vi "UI.vi"() -> ()   [LabVIEW 2015]
panel:
  out "Input Registers 7":u16
  out "Input Registers 6":u16
  out "Input Registers 5":u16
  out "Input Registers 4":u16
  out "Input Registers 3":u16
  out "Input Registers 2":u16
  out "Input Registers 1":u16
  out "Input Registers 0":u16
  in  "Holding Registers 7":u16
  in  "Holding Registers 6":u16
  in  "Holding Registers 5":u16
  in  "Holding Registers 4":u16
  in  "Holding Registers 3":u16
  in  "Holding Registers 2":u16
  in  "Holding Registers 1":u16
  in  "Holding Registers 0":u16
  out "Discrete Inputs 7":bool
  out "Discrete Inputs 6":bool
  out "Discrete Inputs 5":bool
  out "Discrete Inputs 4":bool
  out "Discrete Inputs 3":bool
  out "Discrete Inputs 2":bool
  out "Discrete Inputs 1":bool
  in  "Coils 7":bool
  in  "Coils 6":bool
  in  "Coils 5":bool
  in  "Coils 4":bool
  in  "Coils 3":bool
  in  "Coils 2":bool
  in  "Coils 1":bool
  out "Discrete Inputs 0":bool
  in  "Coils 0":bool
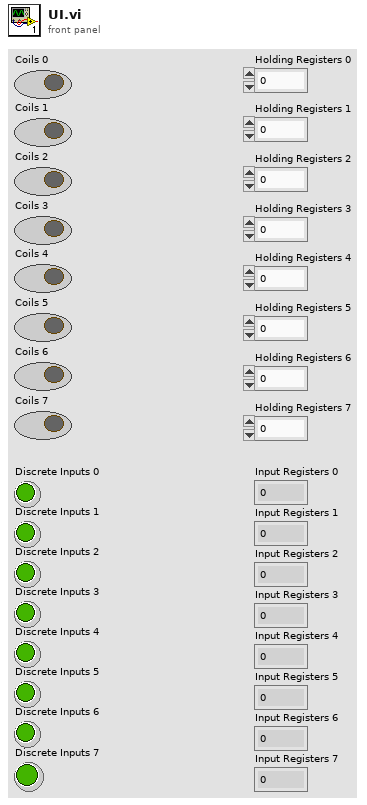
[diagram p1: front panel]
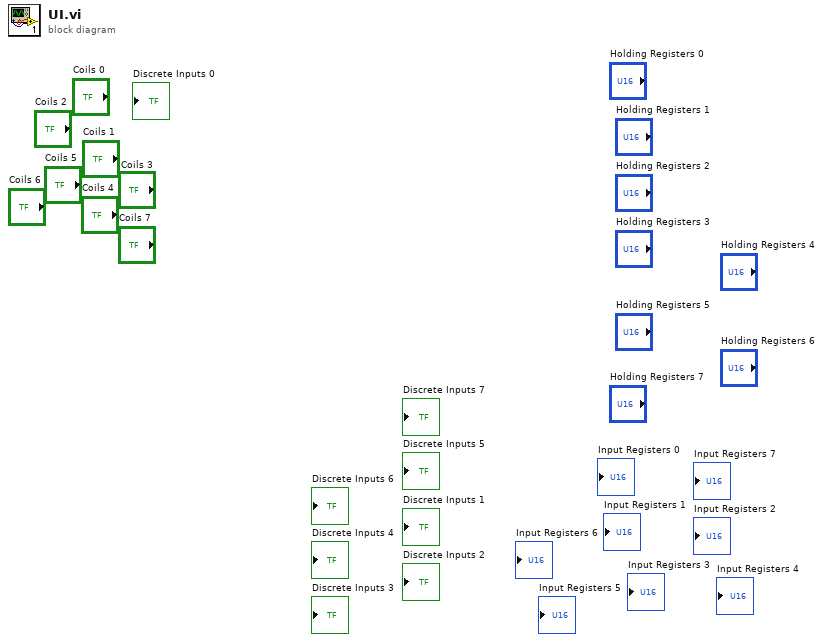
[diagram p0: block diagram]
diagram:
